vi "HRTF-Register Control Events.vi"(7 "Refs":refnum<vi>[](array[refnum]), 11 "error in (no error)":errorcluster) -> (8 "Event Registration Refnum":refnum<event-registration>, 15 "error out":errorcluster)   [LabVIEW 2015]
uses:
  Typedefs/HRTF Config/Events.ctl
  Typedefs/HRTF Config/Selection changed.ctl
  Typedefs/HRTF Config/HRTF Config.xctl
panel:
  in  "temp":cluster{"HRTF Config":T1}
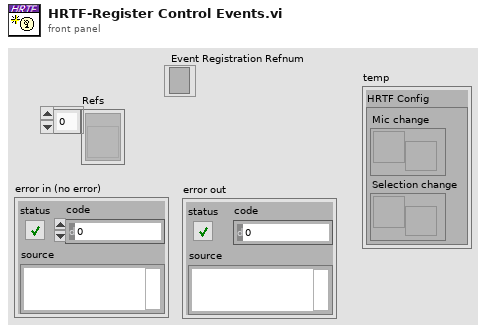
[diagram p1: front panel]
types:
  T1 = typedef "HRTF Config.xctl/Events.ctl" = cluster{"Mic change":refnum<user-event>, "Selection change":refnum<user-event>}
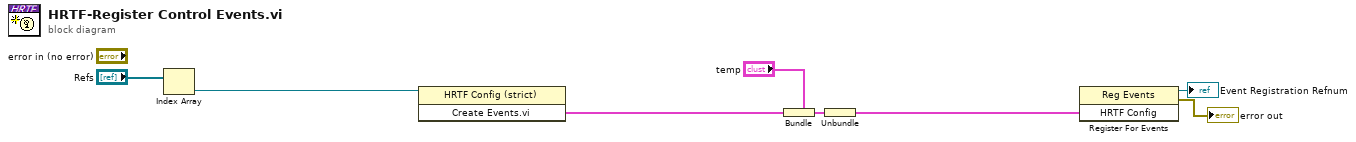
[diagram p0: block diagram]
diagram:
  n1 = Index Array(array="Refs") -> (element=w4:refnum<vi>)  [unwired: 1 in]
  n2 = invoke class="HRTF Config (strict)" method="Create Events.vi"(reference=w4) -> ("Create Events.vi"=w3:T1)  [unwired: 2 in, 2 out]
  n3 = Bundle(cluster="temp", "HRTF Config"=w3) -> (w8:cluster{"HRTF Config":T1})
  n4 = Unbundle(w8) -> ("HRTF Config"=w2:T1)
  n5 = register-events(w2) -> (reference out=→"Event Registration Refnum":refnum<event-registration>, error out=→"error out":errorcluster)  [unwired: 2 in]
